vi "Read Header.vi"(8 "error in":errorcluster, 11 "Path":path=path "C:/Users/kleins/Downloads/CCITT_2.TIF") -> (0 "error out":errorcluster, 1 "IFDOffset":u32, 2 "Tiff Bitness":T1(ring), 3 "refnum out":refnum<file>)   [LabVIEW 2020, in "LV Tiff.lvlib"]
uses:
  LV Tiff.lvlib
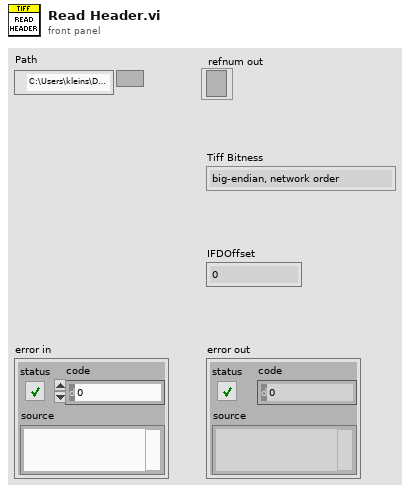
[diagram p1: front panel]
types:
  T1 = enum16{"big-endian, network order", "native, host order", "little-endian"}
  T2 = cluster{"Identifier":u16, "Version":u16, "IFDOffset":u32}
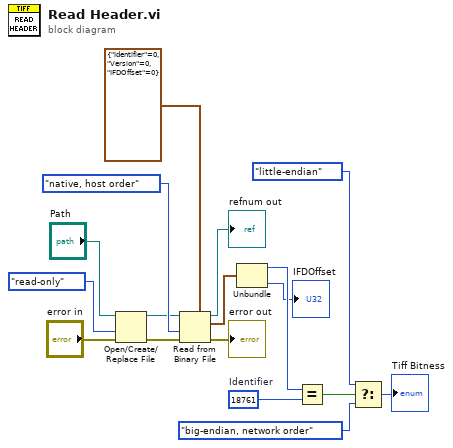
[diagram p0: block diagram]
diagram:
  w14 = u16 18761  # Identifier
  n1 = Open/Create/Replace File(file path (use dialog)="Path", error in="error in", access (0:read/write)=enum16{"read/write", "read-only", "write-only"}."read-only") -> (refnum out=w4:refnum<file>, error out=w2:errorcluster)  [unwired: 3 in, 1 out]
  n2 = Read from Binary File(5:T2 {"Identifier"=0, "Version"=0, "IFDOffset"=0}, 8:w2, 9:T1."native, host order" ("byte order (0:big-endian, network order)"), 11:w4) -> (0:→"error out":errorcluster, 2:w9:T2, 3:→"refnum out":refnum<file>)  [unwired: 2 in, 1 out]
  n3 = Unbundle(w9) -> ("Identifier"=w15:u16, "IFDOffset"=→"IFDOffset":u32)  [unwired: 1 out]
  n4 = Equal?(x=w15, y=w14) -> (x = y?=w13:bool)
  n5 = Select(t=T1."little-endian" ("byte order (0:big-endian, network order)"), s=w13, f=T1."big-endian, network order") -> (s? t:f=→"Tiff Bitness":T1)
